vi "LVClass_HasoField Write HasoField.vi"(8 "error in (no error)":errorcluster, 10 "ClassID_void":T1, 11 "HasoField in":refnum<class "HasoField.lvclass">) -> (0 "error out":errorcluster, 3 "HasoField out":refnum<class "HasoField.lvclass">)   [LabVIEW 2020, in "HasoField.lvclass"]
uses:
  HasoField.lvclass
  Controls/ClassID.ctl
  Controls/Handle creation.ctl
  HasoField.lvclass/HasoField.ctl
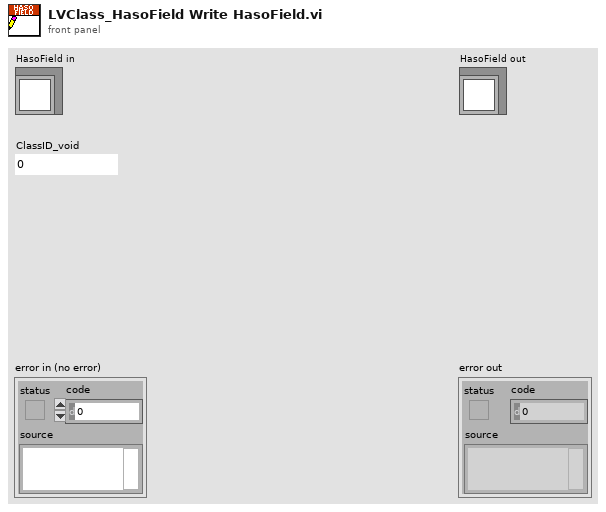
[diagram p1: front panel]
types:
  T1 = typedef "ClassID.ctl" = i64
  T2 = typedef "Handle creation.ctl" = enum16{"By ctor", "By write function"}
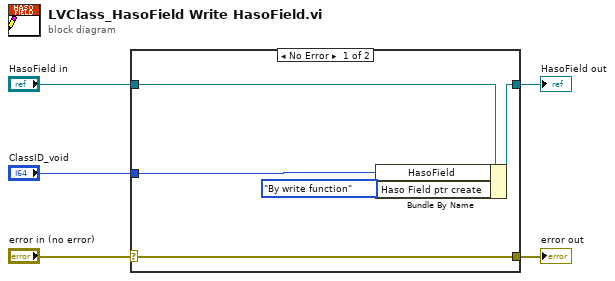
[diagram p0: block diagram]
diagram:
  n1 = case shown="No Error" "error in (no error)" {
    selector: "error in (no error)" -> [w10 w11]
    tunnel: [w10 w11] -> w4
    tunnel: [w8 w12] -> w2
    tunnel: "HasoField in" -> [w9 w12]
    tunnel: "ClassID_void" -> [w7 _]
    frame No Error {
      n2 = Bundle By Name(cluster=w9, "HasoField"=w7, "Haso Field ptr create"=Handle_creation."By write function") -> (w8:refnum<class "HasoField.lvclass">)
    }
    frame Error {
    }
  }
  "error out" <- w4
  "HasoField out" <- w2
